vi "Read Time Stamp of Next.vi"(8 "error in (no error)":errorcluster, 11 "ARecurrence in":refnum<class "ARecurrence.lvclass">) -> (0 "error out":errorcluster, 2 "Time Stamp of Next":timestamp, 3 "ARecurrence out":refnum<class "ARecurrence.lvclass">)   [LabVIEW 2020, in "ARecurrence.lvclass"]
uses:
  ARecurrence.lvclass
  ARecurrence.lvclass/ARecurrence.ctl
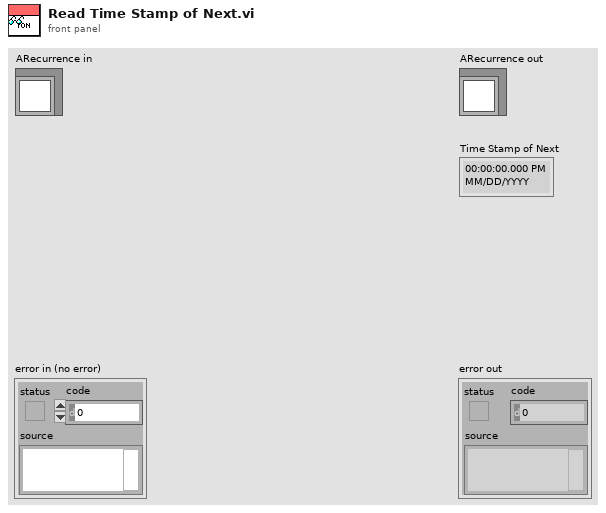
[diagram p1: front panel]
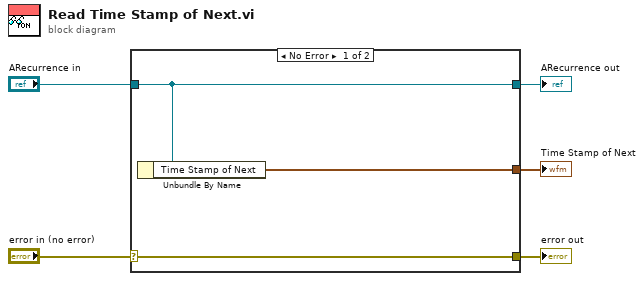
[diagram p0: block diagram]
diagram:
  n1 = case shown="No Error" "error in (no error)" {
    selector: "error in (no error)" -> [w8 w9]
    tunnel: [w8 w9] -> w4
    tunnel: [w7 w10] -> w2
    tunnel: "ARecurrence in" -> [w7 w10]
    tunnel: [w6 _] -> w1
    frame No Error {
      n2 = Unbundle By Name(w7) -> ("Time Stamp of Next"=w6:timestamp)
    }
    frame Error {
    }
  }
  "error out" <- w4
  "ARecurrence out" <- w2
  "Time Stamp of Next" <- w1
